vi "Initialize TCS.vi"(8 "error in (no error)":errorcluster, 9 "TCS COM Port":string="COM1", 10 "TCS Simulated/Real":bool, 11 "SPARC4_GEI in":refnum<class "S4GEI.lvclass">) -> (0 "error out":errorcluster, 3 "SPARC4_GEI out":refnum<class "S4GEI.lvclass">)   [LabVIEW 2018, in "S4GEI.lvclass"]
uses:
  S4GEI.lvclass
  TCS/TCS.lvclass
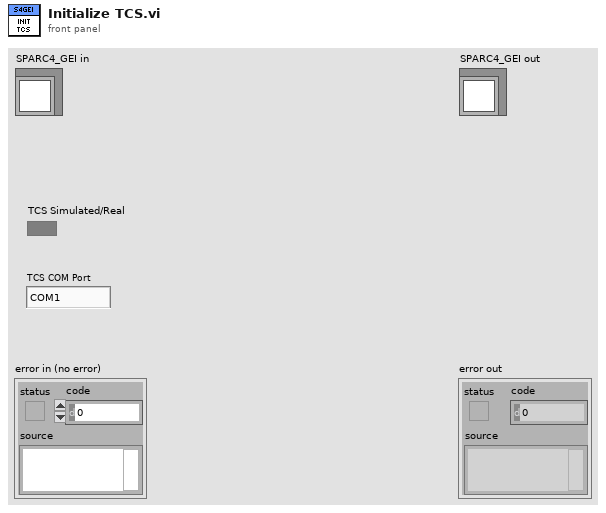
[diagram p1: front panel]
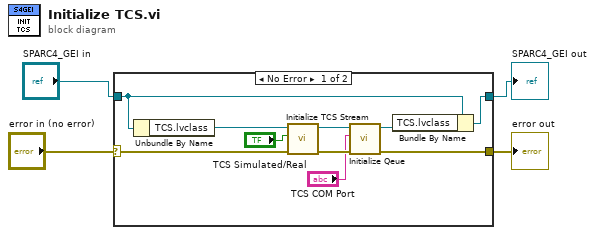
[diagram p0: block diagram]
diagram:
  n1 = case shown="No Error" "error in (no error)" {
    selector: "error in (no error)" -> [w10 w16]
    tunnel: [w7 w16] -> w3
    tunnel: [w14 w15] -> w1
    tunnel: "SPARC4_GEI in" -> [w13 w15]
    frame No Error {
      n2 = Unbundle By Name(w13) -> ("TCS.lvclass"=w9:refnum<class "TCS.lvclass">)
      n3 = call "Initialize TCS Stream.vi"("error in (no error)"=w10, "TCS Simulated/Real"="TCS Simulated/Real", "TCS in"=w9) -> ("error out"=w12:errorcluster, "TCS out"=w11:refnum<class "TCS.lvclass">)  [unwired: 7 in]
      n4 = call "Initialize Qeue.vi"("error in (no error)"=w12, "TCS COM Port"="TCS COM Port", "TCS in"=w11) -> ("error out"=w7:errorcluster, "TCS out"=w8:refnum<class "TCS.lvclass">)  [unwired: 7 in]
      n5 = Bundle By Name(cluster=w13, "TCS.lvclass"=w8) -> (w14:refnum<class "S4GEI.lvclass">)
    }
    frame Error {
    }
  }
  "error out" <- w3
  "SPARC4_GEI out" <- w1
